vi "Strip Quotes From String.vi"(1 "String In":string) -> (0 "Trimmed String":string)   [LabVIEW 2011]
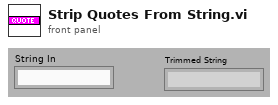
[diagram p1: front panel]
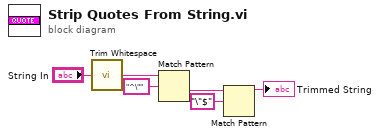
[diagram p0: block diagram]
diagram:
  n1 = call <vilib>:"Trim Whitespace.vi"("string"="String In") -> ("trimmed string"=w1:string)  [unwired: 1 in]
  n2 = Match Pattern(string=w1, regular expression="^\"") -> (after substring=w5:string)  [unwired: 4 out]
  n3 = Match Pattern(string=w5, regular expression="\"$") -> (before substring=→"Trimmed String":string)  [unwired: 4 out]
